vi "CrossHair Hori.vi"(8 "error in (no error)":errorcluster caption="entrée d'erreur (pas d'erreur)", 9 "Couleur Ligne Hori":u32(colorbox)=16770560, 10 "Image In":T1, 11 "Acq Cam Basler en entrée":refnum<class "Acq Cam Basler.lvclass">) -> (0 "error out":errorcluster caption="sortie d'erreur", 2 "Image Out":T1, 3 "Acq Cam Basler en sortie":refnum<class "Acq Cam Basler.lvclass">)   [LabVIEW 2023, in "Acq Cam Basler.lvclass"]
uses:
  Acq Cam Basler.lvclass
  <vilib>/vision/Image Controls.llb/IMAQ Image.ctl
  Acq Cam Basler.lvclass/Acq Cam Basler.ctl
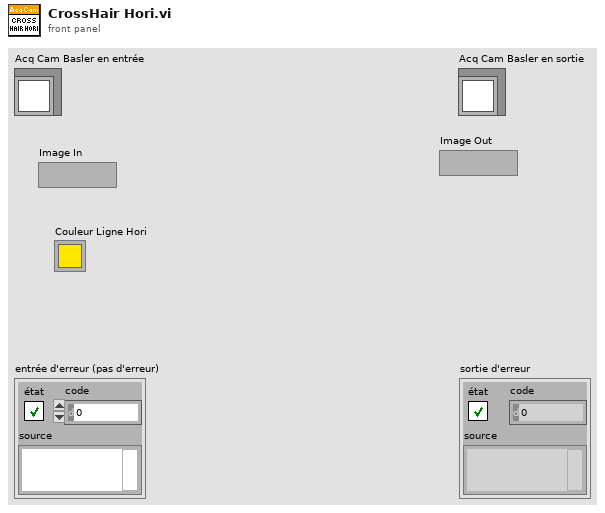
[diagram p1: front panel]
types:
  T1 = typedef "IMAQ Image.ctl" = refnum<image>
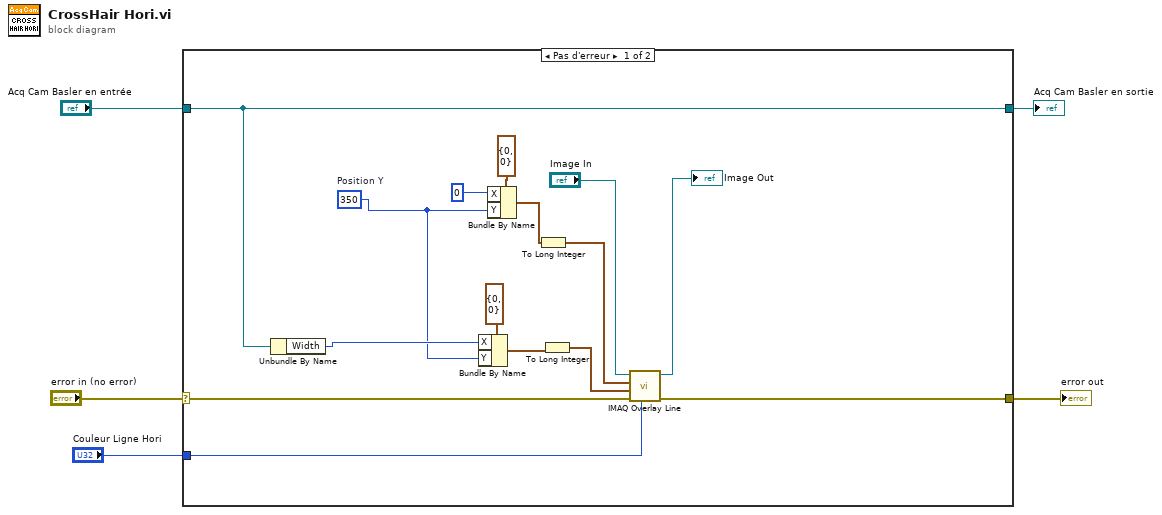
[diagram p0: block diagram]
diagram:
  n1 = case shown="Pas d'erreur" "error in (no error)" {
    selector: "error in (no error)" -> [w14 w22]
    tunnel: [w12 w22] -> w4
    tunnel: [w11 w21] -> w2
    tunnel: "Acq Cam Basler en entrée" -> [w11 w21]
    tunnel: "Couleur Ligne Hori" -> [w13 _]
    frame No Error {
      w6 = u32 350  # Position Y
      n2 = Unbundle By Name(w11) -> ("Width"=w7:u32)
      n3 = Bundle By Name(cluster=cluster{"X":u32, "Y":u32} {"X"=0, "Y"=0} ("End Point"), "X"=w7, "Y"=w6) -> (w19:cluster{"X":u32, "Y":u32})
      n4 = Bundle By Name(cluster=cluster{"X":u32, "Y":u32} {"X"=0, "Y"=0} ("End Point"), "X"=u32 0 ("Y"), "Y"=w6) -> (w20:cluster{"X":u32, "Y":u32})
      n5 = To Long Integer(number=w20) -> (32bit integer=w18:cluster{"X":i32, "Y":i32})
      n6 = To Long Integer(number=w19) -> (32bit integer=w17:cluster{"X":i32, "Y":i32})
      n7 = call "IMAQ Overlay Line"("Color"=w13, "error in (no error)"=w14, "End Point"=w17, "Start Point"=w18, "Image"="Image In") -> ("error out"=w12:errorcluster, "Image Out"=→"Image Out":T1)  [unwired: 1 in, 4 out]
    }
    frame Error {
    }
  }
  "error out" <- w4
  "Acq Cam Basler en sortie" <- w2
